vi "ParseReadValue.vi"(11 "Read Buffer":string) -> (3 "Value":string)   [LabVIEW 2012, in "Sierra-M100.lvlib"]
doc: "This VI gets the value of a \"get\", or \"read\", command."
uses:
  Sierra-M100.lvlib
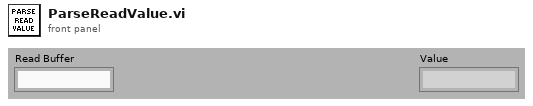
[diagram p1: front panel]
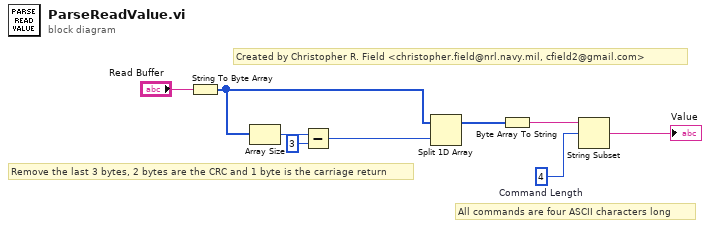
[diagram p0: block diagram]
diagram:
  w2 = 4  # Command Length
  # "Created by Christopher R. Field <christopher.field@nrl.navy.mil, cfield2@gmail.com>"
  # "Remove the last 3 bytes, 2 bytes are the CRC and 1 byte is the carriage return"
  # "All commands are four ASCII characters long"
  n1 = String To Byte Array(string="Read Buffer") -> (unsigned byte array=w8:u8[])
  n2 = Array Size(array=w8) -> (size(s)=w7:i32)
  n3 = Subtract(x=w7, y=3) -> (x-y=w5:i32)
  n4 = Split 1D Array(array=w8, index=w5) -> (first subarray=w4:u8[])  [unwired: 1 out]
  n5 = Byte Array To String(unsigned byte array=w4) -> (string=w3:string)
  n6 = String Subset(string=w3, offset (0)=w2) -> (substring=→"Value":string)  [unwired: 1 in]
